vi "Move_Files.vi"(8 "error in":errorcluster, 9 "Unit Information":string="UnitInformation", 10 "Target Directory to Save U/S Files":path=path "C:/OR/Development Data", 11 "Location of U/S Files":path=path "W:/SRP/TestPrograms/OR_AM3") -> (0 "error out":errorcluster, 2 "Cycle-Cycle-Jitter":string, 3 "Total RMS Jitter":string)   [LabVIEW 2011]
doc: "This VI moves the resultspectrum, resultsweep, and resultxfer from the user specified Testing Directory to the user specified Data directory. This VI also captures the jitter data from the resultspectrum file.\n\nInputs:\n1.Location of U/S Files: The location of the test directory where the SRP will typically save the resultspectrum, resultsweep, and resultxfer files (C:\\SRP\\TestPrograms\\OR_AM3).\n2.Target Directory to Save U/S Files: The location to move the undersampling files. This is typically\nthe data folder (C:\\OR\\Development Data).\n4.Unit Information: Information about the unit which will be appeneded to the U/S file name when moving\nto the new direcotry.\n\nOutputs:\n1. Error: An error has occured.\n2. Total RMS Jitter: The total RMS Jitter as read from the resultspectrum file.\n3. Cycle-Cycle Jitter: The Cycle-Cycle Jitter as read from the result spectrum file."
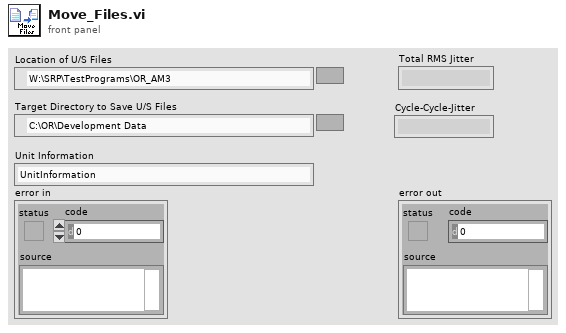
[diagram p1: front panel]
types:
  T1 = enum16{"open", "replace", "create", "open or create", "replace or create", "replace or create with confirmation"}
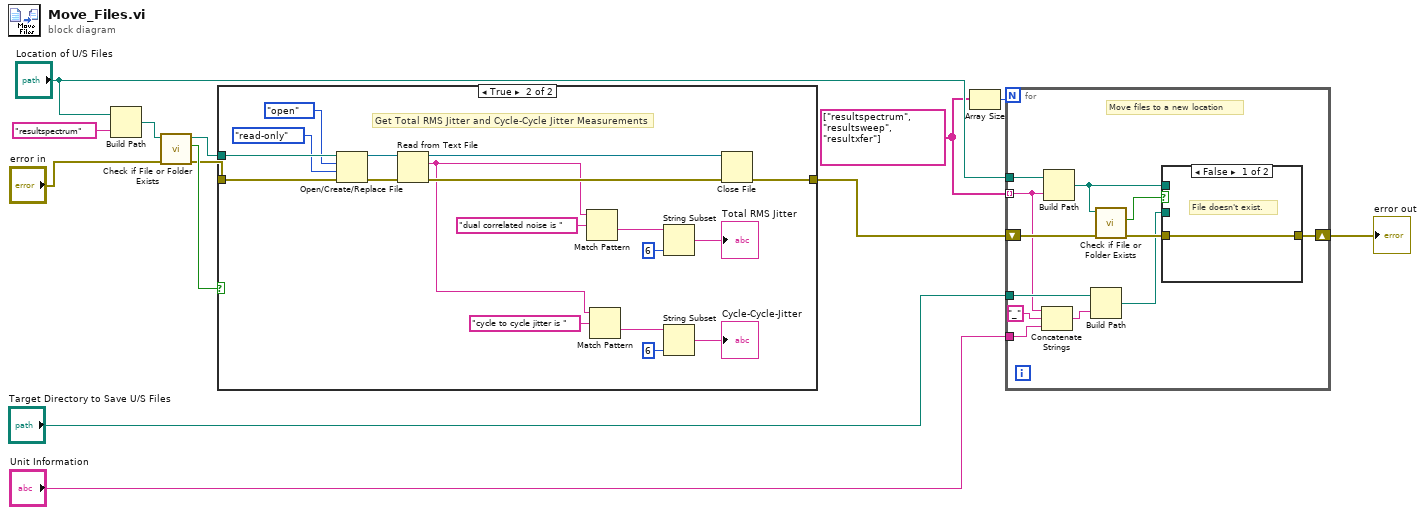
[diagram p0: block diagram]
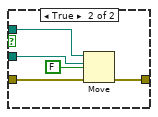
[diagram p2: hidden frame]
diagram:
  w3 = string[] ["resultspectrum", "resultsweep", "resultxfer"]
  n1 = Build Path(base path="Location of U/S Files", name or relative path="resultspectrum") -> (appended path=w8:path)
  n2 = call <vilib>:"Check if File or Folder Exists.vi"("error in (no error)"="error in", "path"=w8) -> ("error out"=w10:errorcluster, "file or folder exists?"=w12:bool, "dup path"=w11:path)  [unwired: 7 in]
  n3 = case shown="True" w12 {
    tunnel: w11 -> [_ w19]
    tunnel: w10 -> [w14 w18]
    tunnel: [w14 w15] -> w6
    frame False {
      # "File doesn't exist."
    }
    frame True {
      # "Get Total RMS Jitter and Cycle-Cycle Jitter Measurements"
      n4 = Open/Create/Replace File(file path (use dialog)=w19, error in=w18, operation (0:open)=T1."open", access (0:read/write)=enum16{"read/write", "read-only", "write-only"}."read-only") -> (refnum out=w21:refnum<file>, error out=w31:errorcluster)  [unwired: 2 in, 1 out]
      n5 = Read from Text File(file (use dialog)=w21, error in=w31) -> (refnum out=w20:refnum<file>, text=w24:string, error out=w32:errorcluster)  [unwired: 2 in, 1 out]
      n6 = Match Pattern(string=w24, regular expression="dual correlated noise is ") -> (after substring=w27:string)  [unwired: 1 in, 3 out]
      n7 = Match Pattern(string=w24, regular expression="cycle to cycle jitter is ") -> (after substring=w28:string)  [unwired: 1 in, 3 out]
      n8 = String Subset(string=w27, length (rest)=6 ("length (rest)")) -> (substring=→"Total RMS Jitter":string)  [unwired: 1 in]
      n9 = String Subset(string=w28, length (rest)=6 ("length (rest)")) -> (substring=→"Cycle-Cycle-Jitter":string)  [unwired: 1 in]
      n10 = Close File(refnum=w20, error in=w32) -> (error out=w15:errorcluster)  [unwired: 1 out]
    }
  }
  n11 = Array Size(array=w3) -> (size(s)=w4:i32)
  n12 = for {
    N: w4 -> [_]
    tunnel: w3 -> [w35] mode=indexing
    tunnel: "Location of U/S Files" -> [w41]
    shift-right: [w39] -> w5
    shift-left: w6 -> [w40]
    tunnel: "Target Directory to Save U/S Files" -> [w37]
    tunnel: "Unit Information" -> [w34]
    # "Move files to a new location"
    n13 = Concatenate Strings(w35, "_" ("string"), w34) -> (w38:string)
    n14 = Build Path(base path=w41, name or relative path=w35) -> (appended path=w44:path)
    n15 = Build Path(base path=w37, name or relative path=w38) -> (appended path=w36:path)
    n16 = call <vilib>:"Check if File or Folder Exists.vi"("error in (no error)"=w40, "path"=w44) -> ("error out"=w43:errorcluster, "file or folder exists?"=w42:bool)  [unwired: 7 in, 1 out]
    n17 = case shown="False" w42 {
      tunnel: w43 -> [w45 w49]
      tunnel: [w45 w48] -> w39
      tunnel: w44 -> [_ w47]
      tunnel: w36 -> [_ w46]
      frame False {
        # "File doesn't exist."
      }
      frame True {
        n18 = Move(source path=w47, error in=w49, 9:FALSE ("overwrite (F)"), 10:w46) -> (error out=w48:errorcluster)  [unwired: 1 in, 2 out]
      }
    }
  }
  "error out" <- w5
